vi "Build One Package.vi"(0 "Destination Path":path, 2 "Build Packge?":bool, 5 "Package Path":path, 7 "Package Spec":string[](array[string]), 11 "error in (no error)":errorcluster) -> (4 "Package Directory":path, 6 "Error Message":string, 15 "error out":errorcluster)   [LabVIEW 2021, in "Measurement Builder.lvlib"]
uses:
  Measurement Builder.lvlib
  Path Functions/Path Functions.lvlib
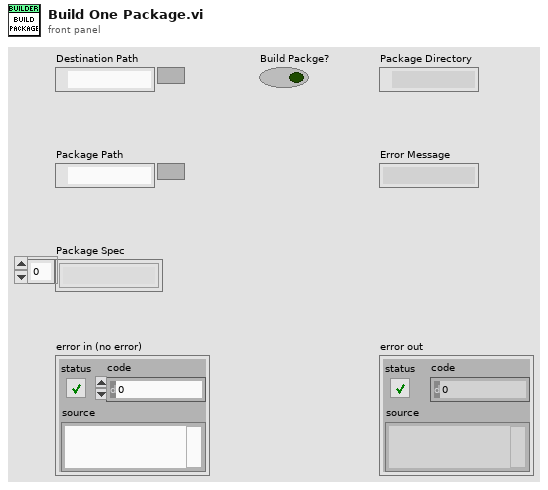
[diagram p1: front panel]
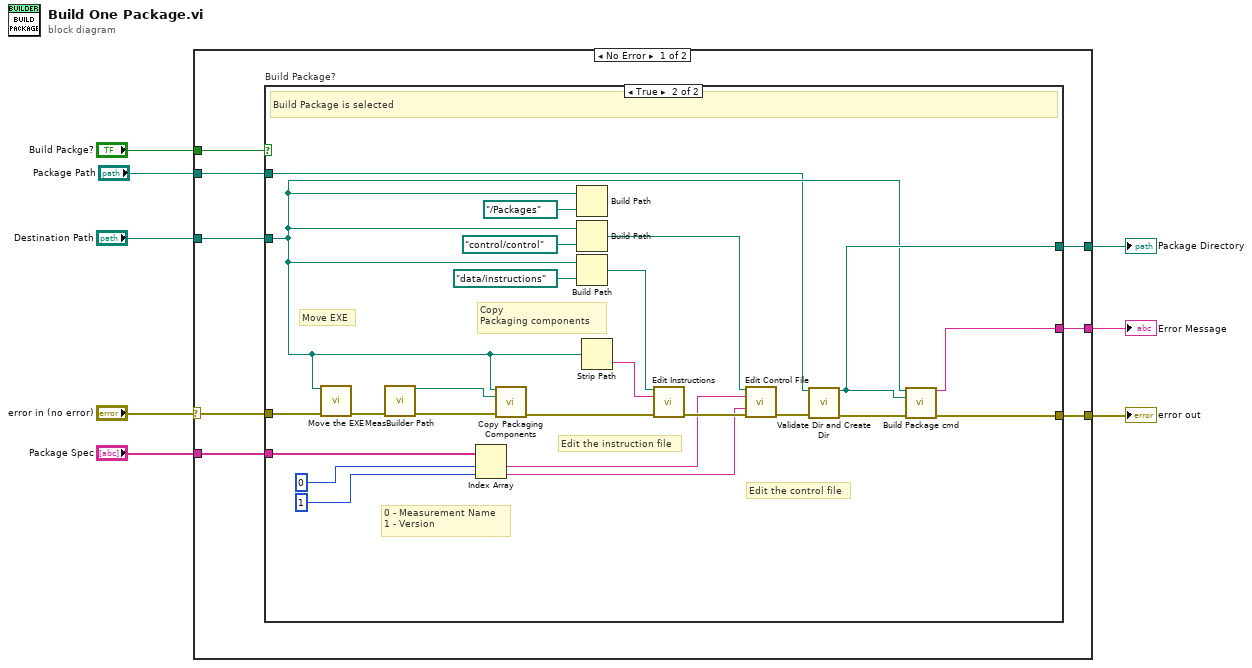
[diagram p0: block diagram]
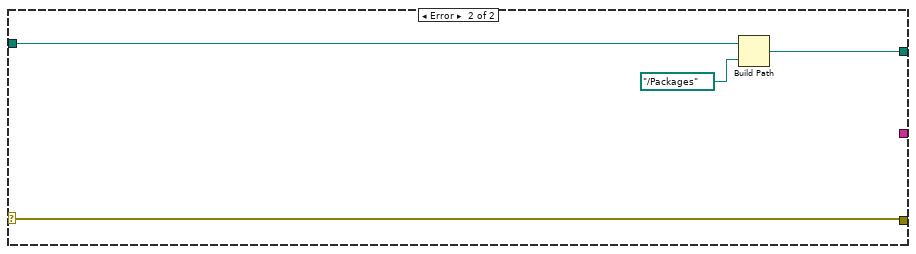
[diagram p3: hidden frame]
diagram:
  n1 = case shown="No Error" "error in (no error)" {
    selector: "error in (no error)" -> [w12 w45]
    tunnel: [w16 w45] -> w8
    tunnel: [w15 w42] -> w7
    tunnel: "Destination Path" -> [w14 w44]
    tunnel: "Package Spec" -> [w13 _]
    tunnel: "Build Packge?" -> [w11 _]
    tunnel: [w10 _] -> w2
    tunnel: "Package Path" -> [w9 _]
    frame No Error {
      n2 = case "Build Package?" shown="True" w11 {
        tunnel: w12 -> [w17 w25]
        tunnel: w13 -> [_ w33]
        tunnel: w14 -> [_ w24]
        tunnel: [_ w30] -> w15
        tunnel: [w17 w26] -> w16
        tunnel: [_ w27] -> w10
        tunnel: w9 -> [_ w18]
        frame False {
        }
        frame True {
          # "Copy \nPackaging components"
          # "Move EXE"
          # "Edit the control file"
          # "Edit the instruction file"
          # "0 - Measurement Name\n1 - Version"
          # "Build Package is selected"
          n3 = call "Move the EXE.vi"("Primary destination path"=w24, "error in (no error)"=w25) -> ("error out"=w21:errorcluster)  [unwired: 13 in]
          n4 = call "MeasBuilder Path.vi"("error in (no error)"=w21) -> ("Template"=w23:path, "error out"=w22:errorcluster)  [unwired: 11 in, 2 out]
          n5 = Index Array(array=w33, index #1=0 ("index"), index #2=1 ("index")) -> (element #1=w19:string, element #2=w20:string)
          n6 = call "Copy Packaging Components.vi"("Primary destination path"=w24, "Template Path"=w23, "error in (no error)"=w22) -> ("error out"=w34:errorcluster)  [unwired: 11 in, 1 out]
          n7 = Build Path(base path=w24, name or relative path=path "../Packages") -> ()  [unwired: 1 out]
          n8 = Build Path(base path=w24, name or relative path=path "control/control") -> (appended path=w28:path)
          n9 = Build Path(base path=w24, name or relative path=path "data/instructions") -> (appended path=w37:path)
          n10 = Strip Path(path=w24) -> (name=w36:string)  [unwired: 1 out]
          n11 = call "Edit Instructions.vi"("Instruction File"=w37, "Meas Name"=w36, "error in (no error)"=w34) -> ("error out"=w38:errorcluster)  [unwired: 12 in]
          n12 = call "Edit Control File.vi"("Control File"=w28, "MeasName"=w19, "Version"=w20, "error in (no error)"=w38) -> ("error out"=w32:errorcluster)  [unwired: 11 in]
          n13 = call "Validate Dir and Create Dir.vi"("Directory"=w18, "error in (no error)"=w32) -> ("Dup Directory"=w30:path, "error out"=w29:errorcluster)  [unwired: 12 in]
          n14 = call "Build Package cmd.vi"("Source Path"=w24, "Destination Dir"=w30, "error in (no error)"=w29) -> ("Error Message"=w27:string, "error out"=w26:errorcluster)  [unwired: 11 in]
        }
      }
    }
    frame Error {
      n15 = Build Path(base path=w44, name or relative path=path "../Packages") -> (appended path=w42:path)
    }
  }
  "error out" <- w8
  "Package Directory" <- w7
  "Error Message" <- w2
